vi "TC200 Control.vi"() -> ()   [LabVIEW 2012]
uses:
  <vilib>/Instr/_visa.llb/Select Event Type.ctl
  <vilib>/Instr/_visa.llb/VISA Configure Serial Port (Instr).vi
  <vilib>/regexp/Match Regular Expression.xnode
panel:
  out "Tset":dbl
  out "T act":dbl
  in  "stop":bool
  out "T vs time":cluster{dbl, dbl}(graph)
  in  "Enable":bool
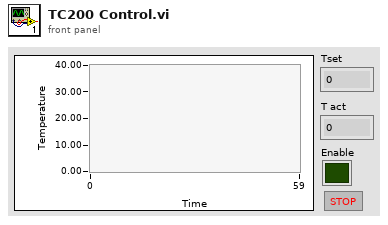
[diagram p1: front panel]
types:
  T1 = typedef "Select Event Type.ctl" = u32
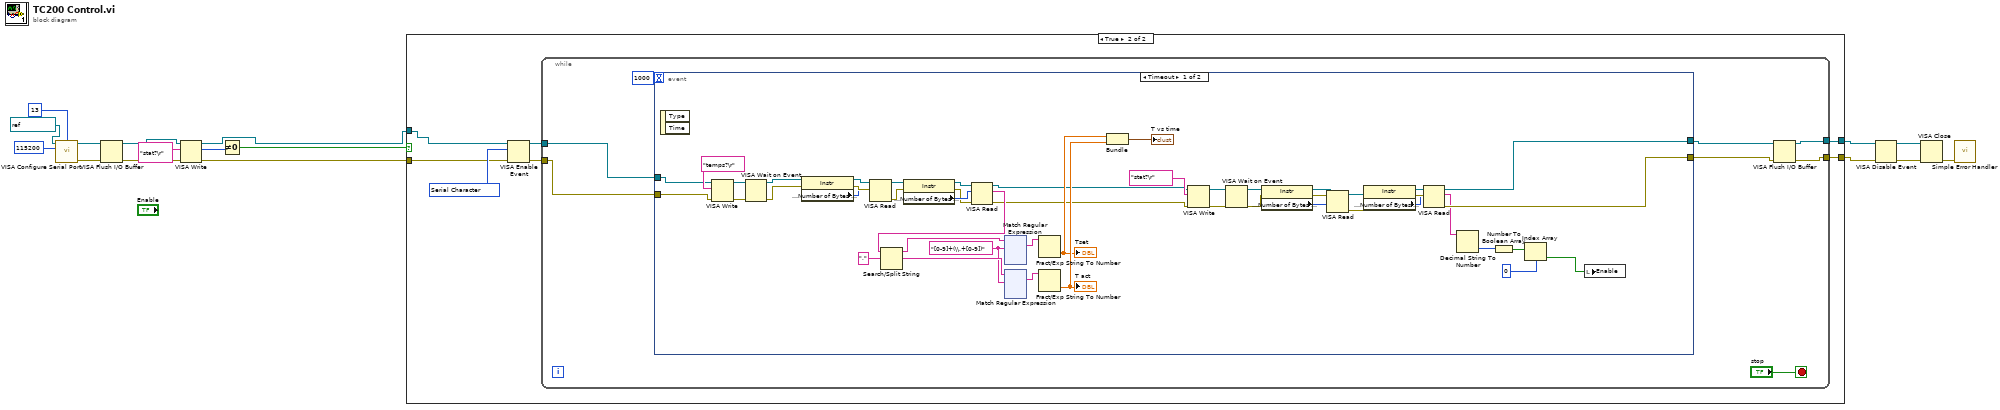
[diagram p0: block diagram]
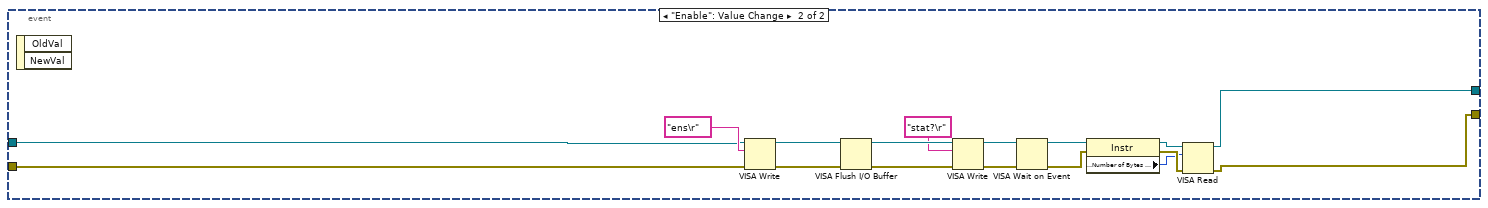
[diagram p3: hidden frame]
diagram:
  n1 = call-poly "VISA Configure Serial Port"("VISA resource name"=refnum<visa-resource-name> "COM2", "termination char\n(0xA = '\\n' = LF)"=u8 13 ("termination char\n(0xA = '\\n' = LF)"), "baud rate (9600)"=u32 115200) -> ("VISA resource name out"=w15:refnum<visa-resource-name>, "error out"=w14:errorcluster)  [unwired: 11 in]
  n2 = VISA Flush I/O Buffer(VISA resource name=w15, error in (no error)=w14) -> (VISA resource name out=w13:refnum<visa-resource-name>, error out=w12:errorcluster)  [unwired: 1 in]
  n3 = VISA Write(VISA resource name=w13, write buffer="stat?\r", error in (no error)=w12) -> (VISA resource name out=w3:refnum<visa-resource-name>, return count=w10:u32, error out=w2:errorcluster)
  n4 = Not Equal To 0?(x=w10) -> (x != 0?=w1:bool)
  n5 = case shown="True" w1 {
    tunnel: w2 -> [w19 w23]
    tunnel: [w18 w26] -> w7
    tunnel: [w19 w25] -> w6
    tunnel: w3 -> [w18 w20]
    frame False {
    }
    frame True {
      w24 = T1 1073684533 items=["Service Request"=1073684491, "Trigger"=3221168138, "Clear"=1073684493, "VXI Signal"=1073684512, "VXI/VME Interrupt"=3221168161, "VXI/VME Sysfail"=1073684509, "VXI/VME Sysreset"=1073684510, "GPIB CIC"=1073684498, "GPIB Talk"=1073684499, "GPIB Listen"=1073684500, "PXI Interrupt"=1073684514, "Serial Break"=1073684515, "Serial TermChar"=1073684516, "Serial CTS"=1073684521, "Serial DSR"=1073684522, "Serial DCD"=1073684524, "Serial RI"=1073684526, "Serial Character"=1073684533, "USB Interrupt"=1073684535, "All Enabled"=1073709055] ("Event Type")
      n6 = VISA Enable Event(8:w23, 10:w24, 11:w20) -> (0:w21:errorcluster, 3:w22:refnum<visa-resource-name>)  [unwired: 1 in]
      n7 = while {
        tunnel: [w30] -> w26
        tunnel: [w29] -> w25
        tunnel: w22 -> [w33]
        tunnel: w21 -> [w32]
        stop <- "stop" stop-if-true
        n8 = event shown="[0] Timeout" {
          selector: _ -> [_ _]
          dyn-events: _ -> [_ _]
          timeout: 1000 -> [_ _]
          tunnel: w33 -> [w58 w319]
          tunnel: w32 -> [w57 w318]
          tunnel: [w41 w312] -> w28
          tunnel: [w40 w311] -> w27
          event Timeout {
            w75 = "[0-9]+(\\.+[0-9])" ("regular expression")
            n9 = event-data() -> ()  [unwired: 1 in, 2 out]
            n10 = VISA Write(VISA resource name=w58, write buffer="temps?\r", error in (no error)=w57) -> (VISA resource name out=w71:refnum<visa-resource-name>, error out=w70:errorcluster)  [unwired: 1 out]
            n11 = VISA Wait on Event(8:w70, 11:w71) -> (0:w68:errorcluster, 3:w67:refnum<visa-resource-name>)  [unwired: 3 in, 2 out]
            n12 = property class="Instr"(reference=w67, error in=w68) -> (reference out=w59:refnum<visa-resource-name>, error out=w61:errorcluster, "Serial Settings:Number of Bytes at Serial Port"=w60:u32)
            n13 = VISA Read(VISA resource name=w59, byte count=w60, error in (no error)=w61) -> (VISA resource name out=w62:refnum<visa-resource-name>, error out=w63:errorcluster)  [unwired: 2 out]
            n14 = property class="Instr"(reference=w62, error in=w63) -> (reference out=w64:refnum<visa-resource-name>, error out=w65:errorcluster, "Serial Settings:Number of Bytes at Serial Port"=w66:u32)
            n15 = VISA Read(VISA resource name=w64, byte count=w66, error in (no error)=w65) -> (VISA resource name out=w43:refnum<visa-resource-name>, read buffer=w72:string, error out=w42:errorcluster)  [unwired: 1 out]
            n16 = Search/Split String(string=w72, search string/char (-)=",") -> (substring before match=w74:string, match + rest of string=w76:string)  [unwired: 1 in, 1 out]
            n17 = xnode "Match Regular Expression"("input string"=w74, "regular expression"=w75) -> ("whole match"=w78:string)  [unwired: 4 in, 4 out]
            n18 = xnode "Match Regular Expression"("input string"=w76, "regular expression"=w75) -> ("whole match"=w77:string)  [unwired: 4 in, 4 out]
            n19 = Fract/Exp String To Number(string=w78) -> (number=w80:dbl)  [unwired: 3 in, 1 out]
            "Tset" <- w80
            n20 = Fract/Exp String To Number(string=w77) -> (number=w81:dbl)  [unwired: 3 in, 1 out]
            "T act" <- w81
            n21 = Bundle(w80, w81) -> (→"T vs time":cluster{dbl, dbl})  [unwired: 1 in]
            n22 = VISA Write(VISA resource name=w43, write buffer="stat?\r", error in (no error)=w42) -> (VISA resource name out=w56:refnum<visa-resource-name>, error out=w55:errorcluster)  [unwired: 1 out]
            n23 = VISA Wait on Event(8:w55, 11:w56) -> (0:w52:errorcluster, 3:w53:refnum<visa-resource-name>)  [unwired: 3 in, 2 out]
            n24 = property class="Instr"(reference=w53, error in=w52) -> (reference out=w51:refnum<visa-resource-name>, error out=w49:errorcluster, "Serial Settings:Number of Bytes at Serial Port"=w50:u32)
            n25 = VISA Read(VISA resource name=w51, byte count=w50, error in (no error)=w49) -> (VISA resource name out=w48:refnum<visa-resource-name>, error out=w47:errorcluster)  [unwired: 2 out]
            n26 = property class="Instr"(reference=w48, error in=w47) -> (reference out=w46:refnum<visa-resource-name>, error out=w45:errorcluster, "Serial Settings:Number of Bytes at Serial Port"=w44:u32)
            n27 = VISA Read(VISA resource name=w46, byte count=w44, error in (no error)=w45) -> (VISA resource name out=w41:refnum<visa-resource-name>, read buffer=w39:string, error out=w40:errorcluster)  [unwired: 1 out]
            n28 = Decimal String To Number(string=w39) -> (number=w38:i32)  [unwired: 2 in, 1 out]
            n29 = Number To Boolean Array(number=w38) -> (Boolean array=w37:bool[])
            n30 = Index Array(array=w37, index=0) -> (element=w35:bool)
            n31 = local write "Enable"(w35) -> ()
          }
          event "Enable": Value Change {
            n32 = event-data() -> ()  [unwired: 1 in, 2 out]
            n33 = VISA Write(VISA resource name=w319, write buffer="ens\r", error in (no error)=w318) -> (VISA resource name out=w305:refnum<visa-resource-name>, error out=w304:errorcluster)  [unwired: 1 out]
            n34 = VISA Flush I/O Buffer(VISA resource name=w305, error in (no error)=w304) -> (VISA resource name out=w317:refnum<visa-resource-name>, error out=w316:errorcluster)  [unwired: 1 in]
            n35 = VISA Write(VISA resource name=w317, write buffer="stat?\r", error in (no error)=w316) -> (VISA resource name out=w309:refnum<visa-resource-name>, error out=w308:errorcluster)  [unwired: 1 out]
            n36 = VISA Wait on Event(8:w308, 11:w309) -> (0:w306:errorcluster, 3:w307:refnum<visa-resource-name>)  [unwired: 3 in, 2 out]
            n37 = property class="Instr"(reference=w307, error in=w306) -> (reference out=w315:refnum<visa-resource-name>, error out=w314:errorcluster, "Serial Settings:Number of Bytes at Serial Port"=w313:u32)
            n38 = VISA Read(VISA resource name=w315, byte count=w313, error in (no error)=w314) -> (VISA resource name out=w312:refnum<visa-resource-name>, error out=w311:errorcluster)  [unwired: 2 out]
          }
        }
        n39 = VISA Flush I/O Buffer(VISA resource name=w28, error in (no error)=w27) -> (VISA resource name out=w30:refnum<visa-resource-name>, error out=w29:errorcluster)  [unwired: 1 in]
      }
    }
  }
  n40 = VISA Disable Event(8:w6, 11:w7) -> (0:w4:errorcluster, 3:w5:refnum<visa-resource-name>)  [unwired: 2 in]
  n41 = VISA Close(VISA resource name=w5, error in (no error)=w4) -> (error out=w8:errorcluster)
  n42 = call <vilib>:"Simple Error Handler.vi"("error in (no error)"=w8) -> ()  [unwired: 1 in, 8 out]
